vi "Search Gateway wrapper.vi"(0 "dwGatewayType":u32, 1 "iLen":i32, 5 "pGWSearchPara":cluster{"dwComIndex":u32, "dwBtr":u32}, 11 "error in (no error)":errorcluster caption="错误输入（无错误）") -> (4 "function return":u32, 6 "pGWSearchPara out":cluster{"dwComIndex":u32, "dwBtr":u32}, 10 "DEV_INFO_OBJ":T1, 15 "error out":errorcluster caption="错误输出")   [LabVIEW 2016, in "UISimCanFunc_wrapper.lvlib"]
doc: "DWORD _declspec(dllexport) SearchGateway_wrapper(DWORD dwGatewayType, P_GW_SEARCH_PARA pGWSearchPara,\n P_DUMMY_DEV_INFO_OBJ pDummy, CHAR pszDevName[64], int iLen);"
uses:
  <userlib>/UISimCanFunc_wrapper/UISimCanFunc_wrapper.lvlib
  <userlib>/UISimCanFunc_wrapper/ctl/DEV_INFO_OBJ.ctl
  <userlib>/UISimCanFunc_wrapper/UISimCanFunc_wrapper.dll
panel:
  in  "pszDevName":string
  in  "pDummy":T2
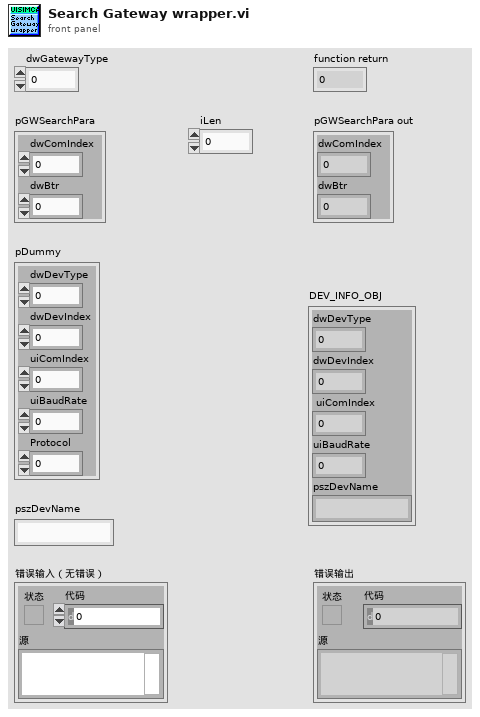
[diagram p1: front panel]
types:
  T1 = typedef "UISimCanFunc_wrapper.lvlib/DEV_INFO_OBJ.ctl" = cluster{"dwDevType":u32, "dwDevIndex":u32, " uiComIndex":u32, "uiBaudRate":u32, "pszDevName":string}
  T2 = cluster{"dwDevType":u32, "dwDevIndex":u32, "uiComIndex":u32, "uiBaudRate":u32, "Protocol":u32}
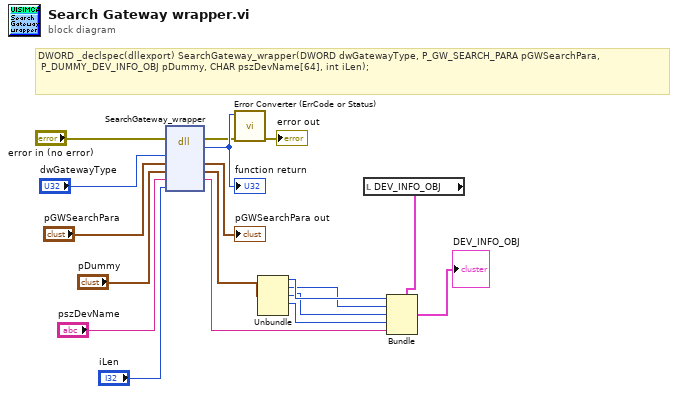
[diagram p0: block diagram]
diagram:
  # "DWORD _declspec(dllexport) SearchGateway_wrapper(DWORD dwGatewayType, P_GW_SEARCH_PARA pGWSearchPara,\n\tP_DUMMY_DEV_INFO_OBJ pDummy, CHAR pszDevName[64], int iLen);"
  n1 = dll-call lib="C:/Program Files (x86)/National Instruments/LabVIEW 2016/user.lib/UISimCanFunc_wrapper/UISimCanFunc_wrapper.*" fn="SearchGateway_wrapper"(error in="error in (no error)", "dwGatewayType"="dwGatewayType", "pGWSearchPara"="pGWSearchPara", "pDummy"="pDummy", "pszDevName"="pszDevName", "iLen"="iLen") -> (error out=w10:errorcluster, w18:u32, "pGWSearchPara"=→"pGWSearchPara out":cluster{"dwComIndex":u32, "dwBtr":u32}, "pDummy"=w5:T2, "pszDevName"=w6:string)  [unwired: 4 in, 1 out]
  "function return" <- w18
  n2 = call <userlib>:"Error Converter (ErrCode or Status).vi"("error in (no error)"=w10, "error code"=w18) -> ("error out"=→"error out":errorcluster)  [unwired: 9 in]
  n3 = Unbundle(w5) -> ("dwDevType"=w4:u32, "dwDevIndex"=w3:u32, "uiComIndex"=w2:u32, "uiBaudRate"=w1:u32)  [unwired: 1 out]
  n4 = local read "DEV_INFO_OBJ"() -> (w8:T1)
  n5 = Bundle(cluster=w8, "dwDevType"=w4, "dwDevIndex"=w3, "uiComIndex"=w2, "uiBaudRate"=w1, "pszDevName"=w6) -> (→"DEV_INFO_OBJ":T1)
